vi "process.vi"(6 "# rolling average":i32, 7 "extra offset":dbl=10.0, 8 "error out 2":errorcluster, 9 "# lines to skip":i32, 10 "# subpatterns":i32, 11 "images":refnum<class "Image.lvclass">[](array[class])) -> (0 "error out":errorcluster, 3 "Array":dbl[][](array[numeric]))   [LabVIEW 2010, in "AnalysisRaps2.lvclass"]
uses:
  AnalysisRaps2.lvclass
  common/classes/Image/Image/Image.lvclass
panel:
  out "min value":dbl
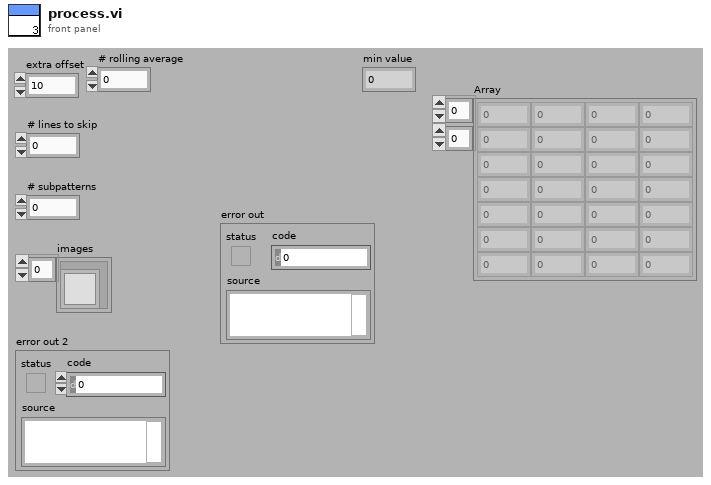
[diagram p1: front panel]
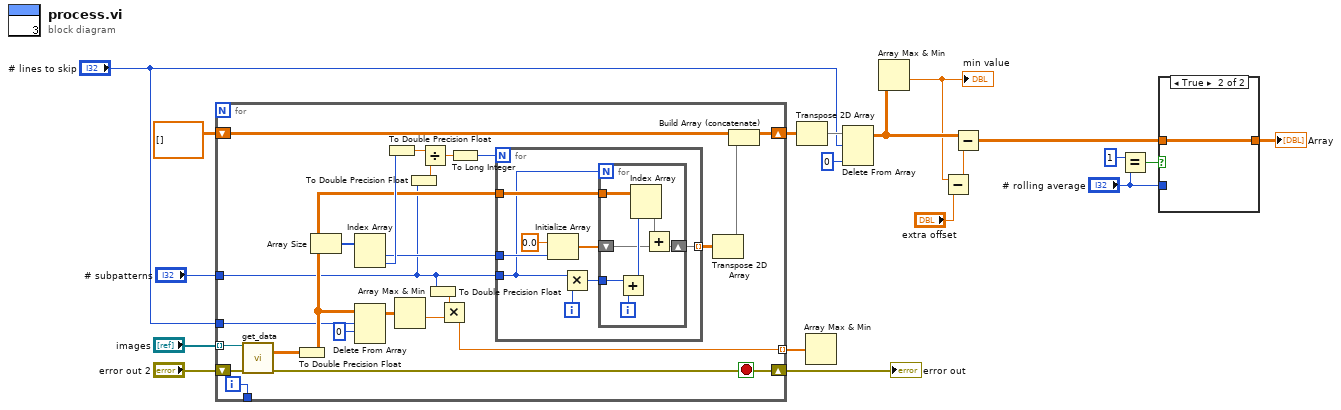
[diagram p0: block diagram]
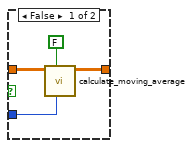
[diagram p2: hidden frame]
diagram:
  n1 = for {
    tunnel: "images" -> [w42] mode=indexing
    shift-right: [w30] -> w16
    shift-left: "error out 2" -> [w43]
    tunnel: "# subpatterns" -> [w23]
    shift-right: [w31] -> w17
    shift-left: dbl[][] [] ("transposed array") -> [w33]
    tunnel: [w28] -> _
    tunnel: "# lines to skip" -> [w25]
    tunnel: [w20] -> w8 mode=indexing
    i -> [w28]
    stop <- w30 stop-if-true
    n2 = call-dynamic "get_data.vi"("Image in"=w42, "error in (no error)"=w43) -> ("Image Pixels (Float)"=w29:sgl[][], "error out"=w30:errorcluster)  [unwired: 5 in, 7 out]
    n3 = To Double Precision Float(number=w29) -> (double precision float=w27:dbl[][])
    n4 = Array Size(array=w27) -> (size(s)=w35:i32[])
    n5 = Index Array(array=w35) -> (element #1=w36:i32, element #2=w37:i32)  [unwired: 2 in]
    n6 = Delete From Array(array=w27, length=w25, index (row)=0) -> (array with subset deleted=w24:dbl[][])  [unwired: 1 in, 1 out]
    n7 = To Double Precision Float(number=w37) -> (double precision float=w39:dbl)
    n8 = Array Max & Min(array=w24) -> (min value=w21:dbl)  [unwired: 3 out]
    n9 = To Double Precision Float(number=w23) -> (double precision float=w40:dbl)
    n10 = Divide(x=w39, y=w40) -> (x/y=w38:dbl)
    n11 = To Double Precision Float(number=w23) -> (double precision float=w22:dbl)
    n12 = Multiply(x=w22, y=w21) -> (x*y=w20:dbl)
    n13 = To Long Integer(number=w38) -> (32bit integer=w41:i32)
    n14 = for {
      N: w41 -> [_]
      tunnel: w27 -> [w51]
      tunnel: w23 -> [w44]
      tunnel: [w48] -> w34 mode=indexing
      tunnel: w36 -> [w46]
      i -> [w50]
      n15 = Initialize Array(0.0, w46) -> (w45:dbl[])
      n16 = Multiply(x=w44, y=w50) -> (x*y=w49:i32)
      n17 = for {
        N: w44 -> [_]
        tunnel: w51 -> [w58]
        tunnel: w49 -> [w56]
        shift-right: [w53] -> w48
        shift-left: w45 -> [w52]
        i -> [w57]
        n18 = Add(x=w56, y=w57) -> (x+y=w55:i32)
        n19 = Index Array(array=w58, index (col)=w55) -> (element=w54:dbl[])  [unwired: 1 in]
        n20 = Add(x=w54, y=w52) -> (x+y=w53:dbl[])
      }
    }
    n21 = Transpose 2D Array(2D array=w34) -> (transposed array=w32:dbl[][])
    n22 = Build Array (concatenate)(w33, w32) -> (w31:dbl[][])
  }
  "error out" <- w16
  n23 = Transpose 2D Array(2D array=w17) -> (transposed array=w18:dbl[][])
  n24 = Array Max & Min(array=w8) -> ()  [unwired: 4 out]
  n25 = Delete From Array(array=w18, length="# lines to skip", index (col)=0 ("disabled index (col)")) -> (array with subset deleted=w7:dbl[][])  [unwired: 1 in, 1 out]
  n26 = Array Max & Min(array=w7) -> (min value=w6:dbl)  [unwired: 3 out]
  "min value" <- w6
  n27 = Subtract(x=w6, y="extra offset") -> (x-y=w12:dbl)
  n28 = Subtract(x=w7, y=w12) -> (x-y=w5:dbl[][])
  n29 = Equal?(x=1 ("y"), y="# rolling average") -> (x = y?=w1:bool)
  n30 = case shown="True" w1 {
    tunnel: w5 -> [w62 w63]
    tunnel: [w61 w63] -> w4
    tunnel: "# rolling average" -> [w59 _]
    frame False {
      n31 = call "calculate_moving_average.vi"("dimension size"=w59, "vertical? (N)"=FALSE ("vertical? (Y)"), "array in"=w62) -> ("array out"=w61:dbl[][])  [unwired: 8 in]
    }
    frame True {
    }
  }
  "Array" <- w4
